vi "live view D05.vi"() -> ()   [LabVIEW 2019, in "D05.lvlib"]
uses:
  D05.lvlib
  <vilib>/userDefined/High Color/IMAQdx.ctl
  <vilib>/vision/Image Controls.llb/IMAQ Image.ctl
  <vilib>/measure/mamon.llb/Trigger Detection for 1 Channel.vi
  <vilib>/measure/NI_MAPro.lvlib
  Calibration Lib.lvlib
  database.lvlib
  <vilib>/vision/driver/NI_Vision_Acquisition_Software.lvlib
panel:
  out "Error out":errorcluster
  in  "Save Button":bool
  in  "Calib IMQ Num":u16(ring) items=["First IMQ", "Second IMQ", "Third IMQ"]
  in  "Verify Calibration1 D05":bool caption="capture grab"
  in  "snapshot":bool
  out "error prj04":errorcluster
  in  "Verify Calibration D05":bool caption="capture grab"
  in  "Close":bool
  in  "Method 2 save D05":bool caption="capture grab"
  in  "Method 1 Save D05":bool caption="Saving txt"
  out "Average Result":string="Average Result"
  out ">18  A":dbl(slide)=1.0 caption=">16 mm" scale=0.0..100.0
  out "16-18  A":dbl(slide)=1.0 caption="14-16 mm" scale=0.0..100.0
  out "14-16  A":dbl(slide)=1.0 caption="12.7-14 mm" scale=0.0..100.0
  out "12.5-14 A":dbl(slide)=1.0 caption="11-12.7 mm" scale=0.0..100.0
  out "10-12.5  A":dbl(slide)=1.0 caption="9.5-11 mm" scale=0.0..100.0 scale format="%#_4f"
  out "8-10  A":dbl(slide)=1.0 caption="8-9.5 mm" scale=0.0..100.0
  out "6.3-8  A":dbl(slide)=1.0 caption="6.3-8 mm" scale=0.0..100.0
  out "<6.3  A":dbl(slide)=1.0 caption="<6.3 mm" scale=0.0..100.0
  out "Live Result":string="Live Result"
  out ">18  L":dbl(slide)=1.0 caption=">16 mm" scale=0.0..100.0
  out "Live View":T1(plugin-control) caption="Disc 26"
  out "16-18  L":dbl(slide)=1.0 caption="14-16 mm" scale=0.0..100.0
  out "14-16  L":dbl(slide)=1.0 caption="12.7-14 mm" scale=0.0..100.0
  out "12.5-14 L":dbl(slide)=1.0 caption="11-12.7 mm" scale=0.0..100.0
  out "10-12.5  L":dbl(slide)=1.0 caption="9.5-11 mm" scale=0.0..100.0 scale format="%#_4f"
  out "8-10  L":dbl(slide)=1.0 caption="8-9.5 mm" scale=0.0..100.0
  out "6.3-8  L":dbl(slide)=1.0 caption="6.3-8 mm" scale=0.0..100.0
  out "<6.3  L":dbl(slide)=1.0 caption="<6.3 mm" scale=0.0..100.0
  out "disc name":string="Live Info Disc 05"
  out "dsgs":string="DSGS"
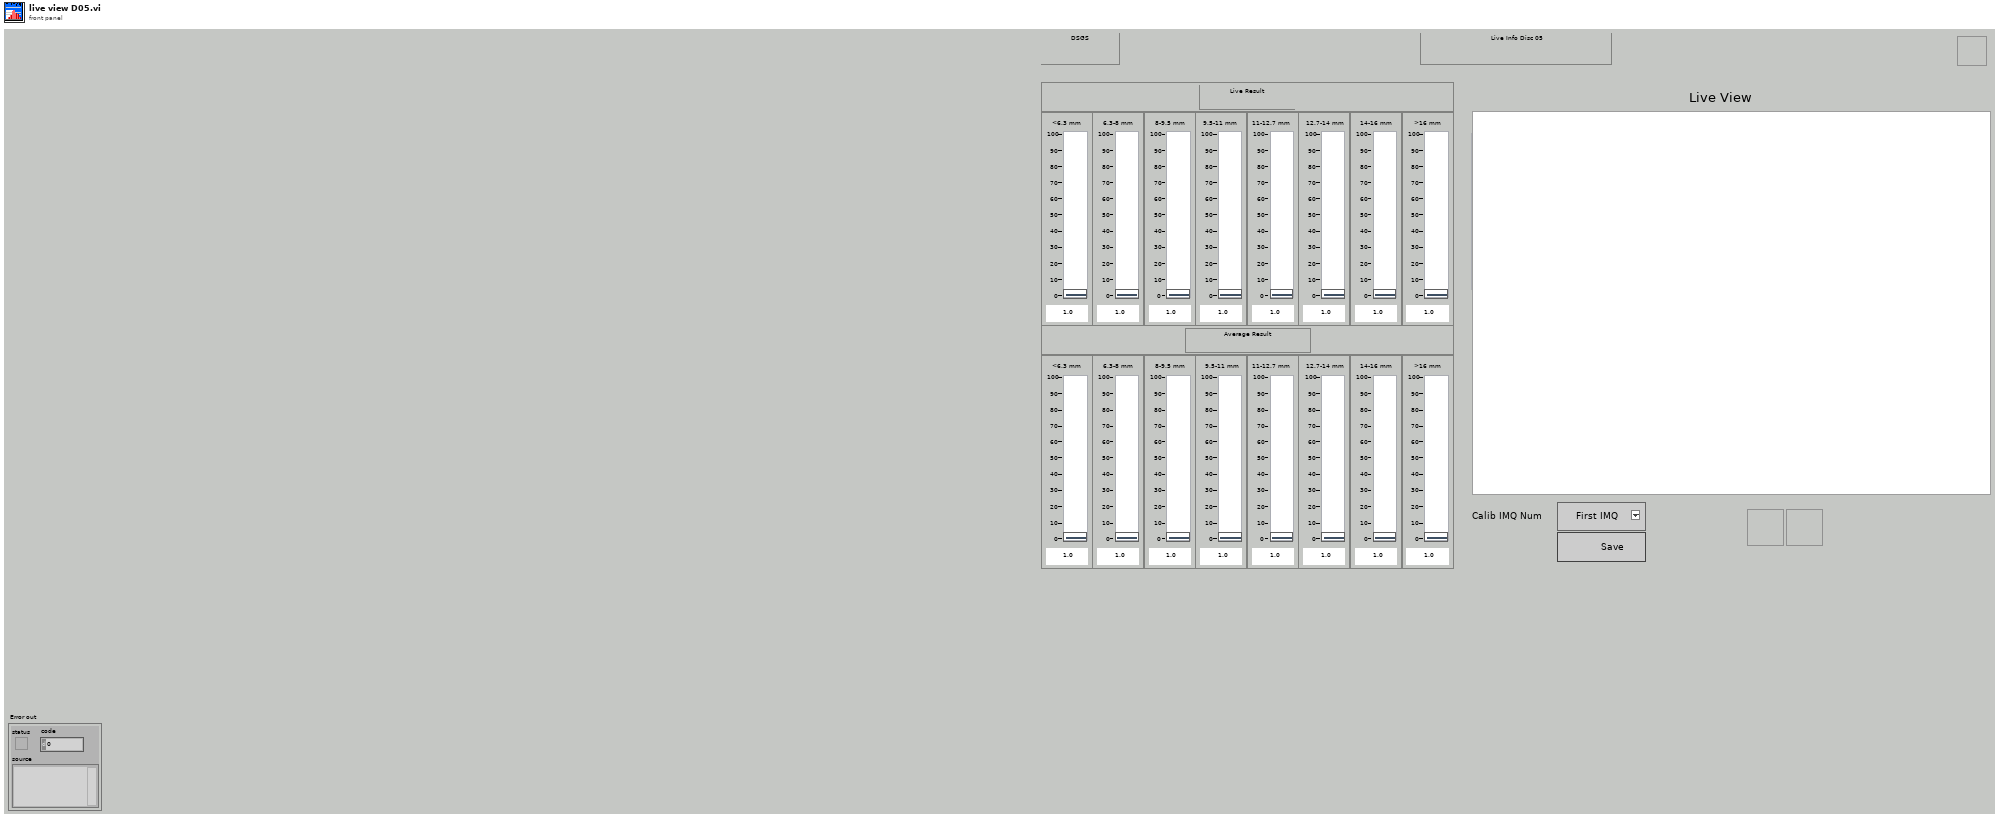
[diagram p1: front panel]
types:
  T1 = typedef "IMAQ Image.ctl" = refnum<image>
  T2 = typedef "IMAQdx.ctl" = refnum<k21>
  T3 = enum8{"Enabled", "Disabled", "Disabled and Grayed Out"}
  T4 = cluster{"date/time string":string, "date/time string":string, string, "Value":dbl, "Value":dbl, "Value":dbl, "Value":dbl, "Value":dbl, "Value":dbl, "Value":dbl, "Value":dbl}
  T5 = cluster{"date/time string":string, "date/time string":string, i32, "spreadsheet string":string, "spreadsheet string":string}
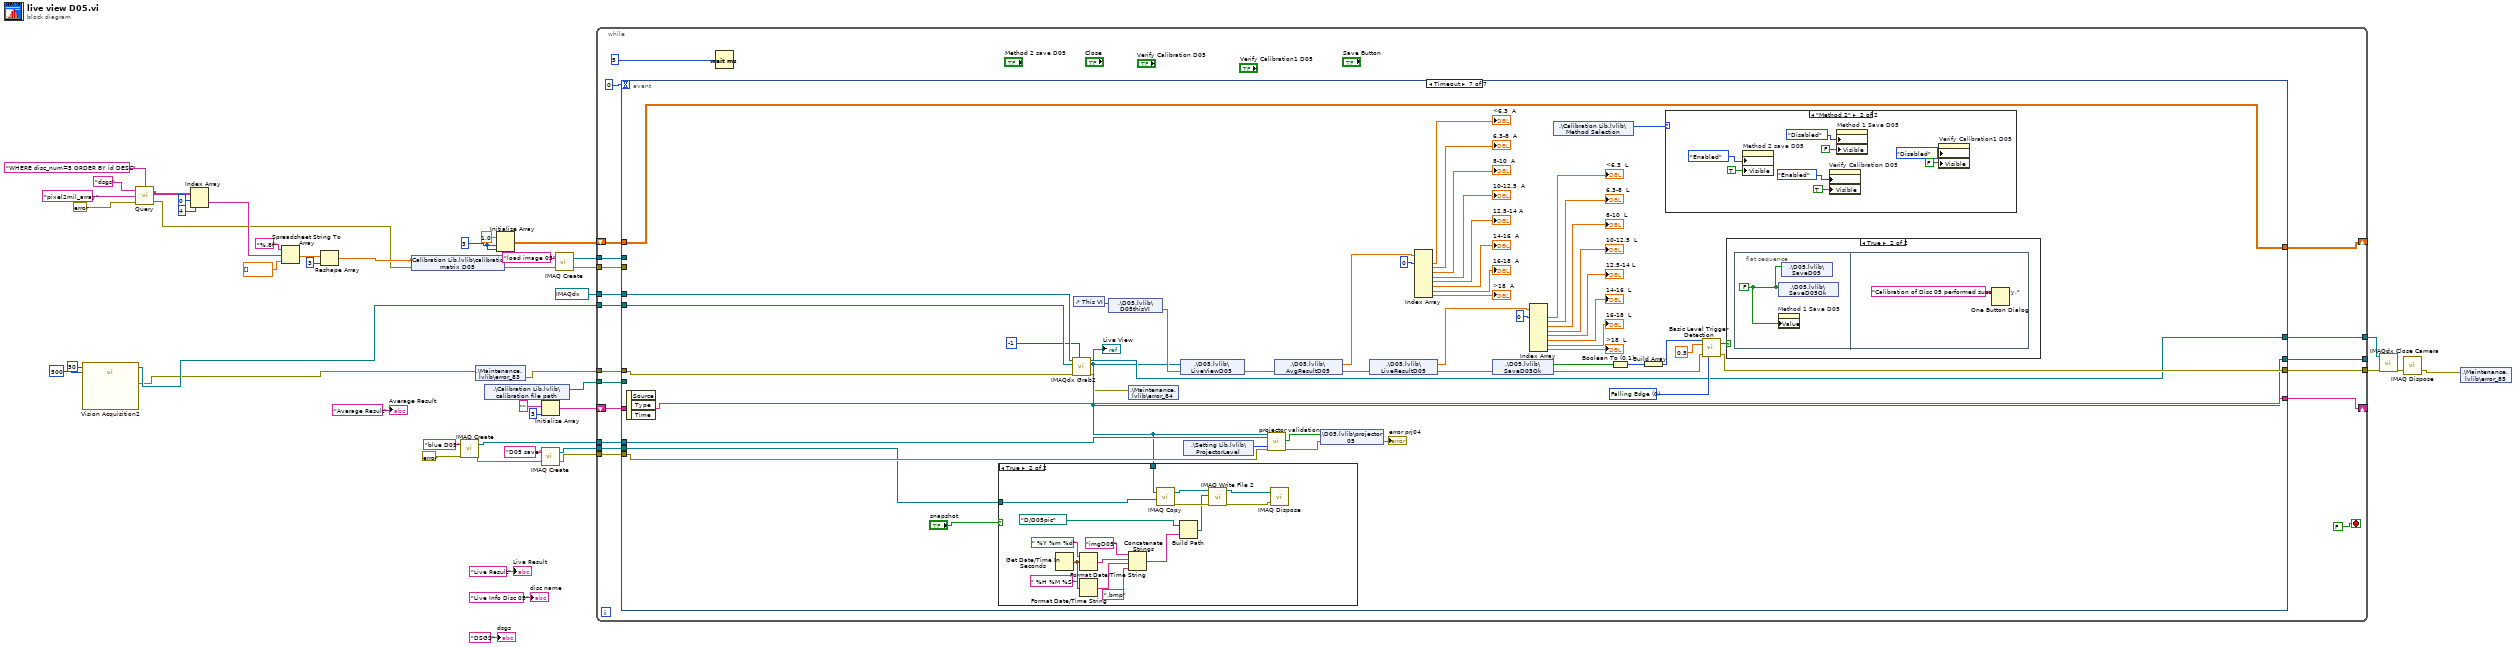
[diagram p0: block diagram]
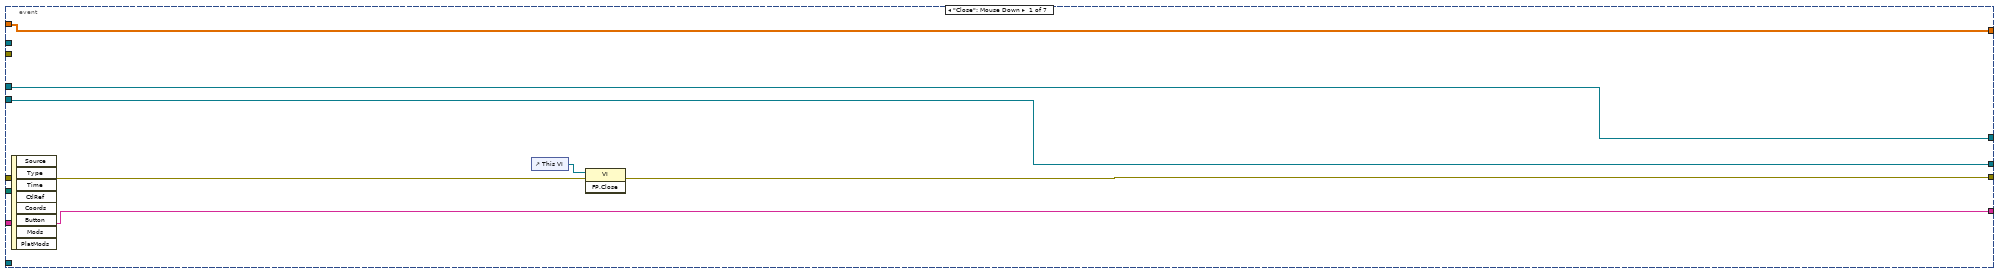
[diagram p2: hidden frame]
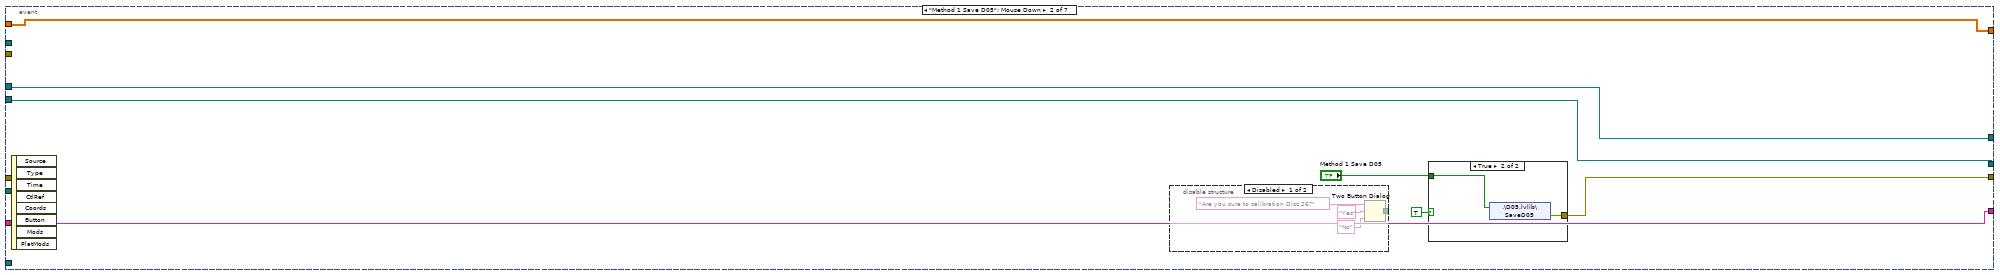
[diagram p3: hidden frame]
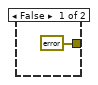
[diagram p5: hidden frame]
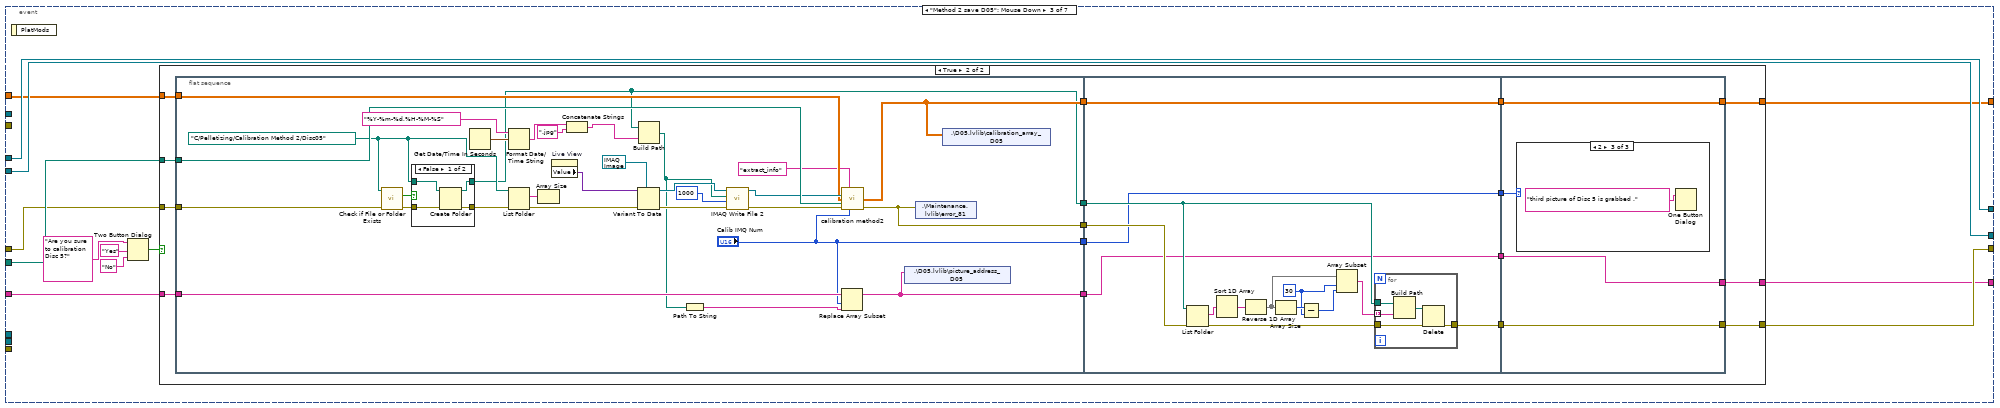
[diagram p6: hidden frame]
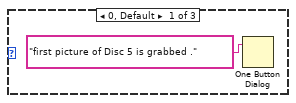
[diagram p9: hidden frame]
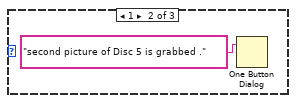
[diagram p10: hidden frame]
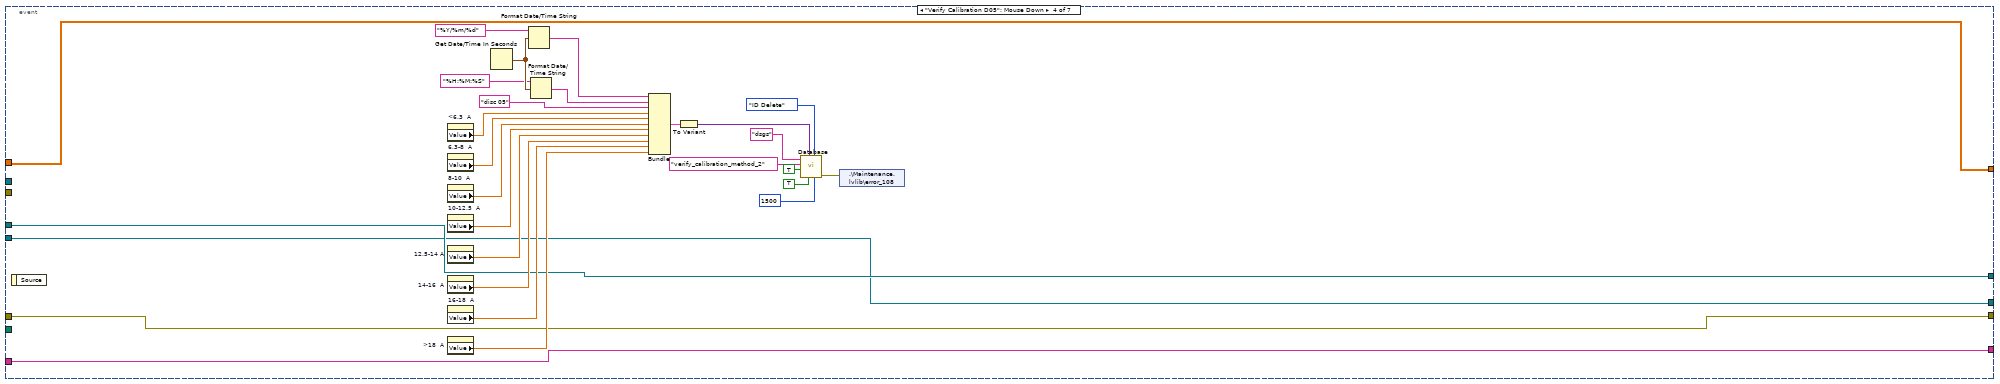
[diagram p11: hidden frame]
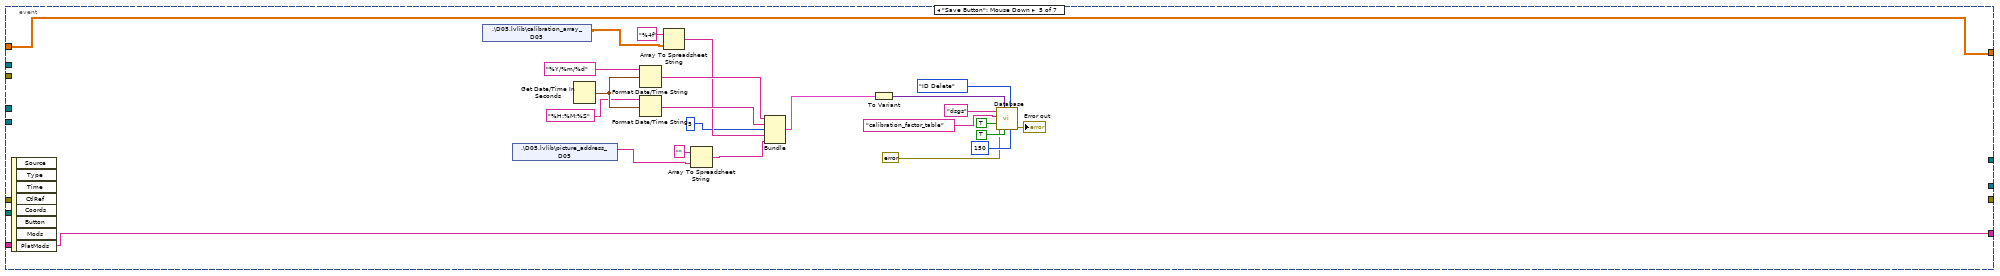
[diagram p12: hidden frame]
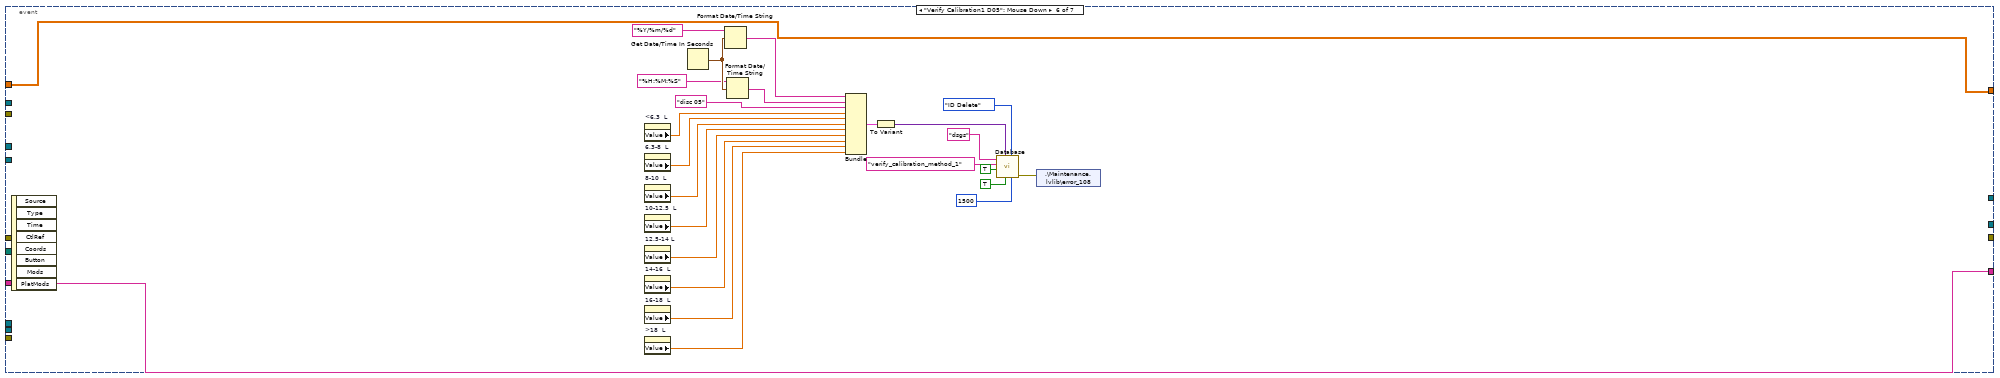
[diagram p13: hidden frame]
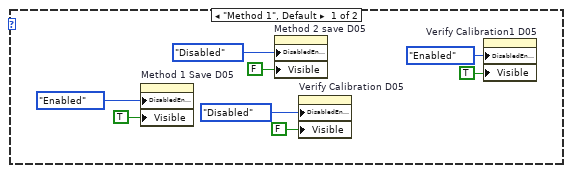
[diagram p15: hidden frame]
diagram:
  w15 = 3 ("dimension size")
  n1 = call "Vision Acquisition2"("Gain (Raw)"=i64 50, "Exposure Time (Raw)"=i64 500) -> ("Image Out"=w4:T1, "error out"=w3:errorcluster)  [unwired: 23 in, 1 out]
  n2 = call "Query.vi"("Condition"="WHERE disc_num=5 ORDER BY id DESC", "Error in"=errorcluster {"status"=FALSE, "code"=0, "source"=""}, "Table Name"="pixel2mil_array", "Connection Name"="dsgs") -> ("Error out"=w7:errorcluster, "data"=w10:string[][])
  n3 = Index Array(array=w10, index (row)=0, index (col)=4 ("disabled index (col)")) -> (element=w8:string)
  n4 = Spreadsheet String To Array(format string="%.8f", spreadsheet string=w8, array type (2D Dbl)=sgl[] []) -> (array=w28:sgl[])  [unwired: 1 in]
  n5 = Reshape Array(w28, 3 ("dimension size")) -> (w25:sgl[])
  n6 = shared-variable ".\\Calibration Lib.lvlib\\calibration matrix D05"(w25, error in=w7) -> (error out=w24:errorcluster)
  n7 = call "IMAQ Create"("Image Name"="blue D05", "error in (no error)"=errorcluster {"status"=FALSE, "code"=0, "source"=""}) -> ("New Image"=w22:T1, "error out"=w20:errorcluster)  [unwired: 3 in]
  n8 = shared-variable ".\\Maintenance.lvlib\\error_83"(w3) -> (error out=w37:errorcluster)  [unwired: 1 in]
  n9 = shared-variable ".\\Calibration Lib.lvlib\\calibration file path"() -> (w38:path)  [unwired: 1 in, 1 out]
  n10 = Initialize Array(1.0 ("element"), w15, w15) -> (w14:dbl[][])
  n11 = call "IMAQ Create"("Image Name"="D05 save", "error in (no error)"=w20) -> ("New Image"=w17:T1, "error out"=w19:errorcluster)  [unwired: 3 in]
  n12 = Initialize Array("", 3 ("dimension size")) -> (w11:string[])
  n13 = call "IMAQ Create"("Image Name"="load image 05", "error in (no error)"=w24) -> ("New Image"=w34:T1, "error out"=w35:errorcluster)  [unwired: 3 in]
  n14 = while {
    tunnel: w38 -> [w63]
    tunnel: w37 -> [w62]
    tunnel: w4 -> [w60]
    tunnel: [w59] -> w42
    tunnel: [w58] -> _
    tunnel: T2 "cam4" ("Session In") -> [w57]
    tunnel: [w56] -> w39
    tunnel: w35 -> [w55]
    tunnel: w34 -> [w54]
    tunnel: w22 -> [w53]
    tunnel: w19 -> [w52]
    tunnel: w17 -> [w51]
    shift-right: [w49] -> _
    shift-left: w14 -> [w50]
    shift-right: [w47] -> _
    shift-left: w11 -> [w48]
    stop <- FALSE stop-if-true
    n15 = event shown="[6] Timeout" {
      selector: _ -> [_ _ _ _ _ _ _]
      dyn-events: _ -> [_ _ _ _ _ _ _]
      timeout: 0 -> [_ _ _ _ _ _ _]
      tunnel: w63 -> [_ _ w99 _ _ _ _]
      tunnel: [w71 w79 w95 w187 _ _ w276] -> w59
      tunnel: w62 -> [w70 _ w98 w187 _ _ w259]
      tunnel: w60 -> [w69 w78 w97 w185 _ _ w264]
      tunnel: [w69 w78 w97 w185 _ _ w261] -> w58
      tunnel: w57 -> [w68 w77 w96 w186 _ _ w263]
      tunnel: [w68 w77 w96 w186 _ _ w262] -> w56
      tunnel: w55 -> [_ _ _ _ _ _ _]
      tunnel: w54 -> [_ _ _ _ _ _ _]
      tunnel: w53 -> [_ _ _ _ _ _ w274]
      tunnel: w52 -> [_ _ _ _ _ _ w270]
      tunnel: w51 -> [_ _ _ _ _ _ w267]
      tunnel: w50 -> [w67 w74 w90 w182 w211 w234 w266]
      tunnel: [w67 w74 w89 w182 w211 w234 w266] -> w49
      tunnel: w48 -> [w66 w73 w88 w181 w210 w233 w265]
      tunnel: [w66 w73 w87 w181 w210 w233 w265] -> w47
      event "Close": Mouse Down {
        n16 = event-data() -> ()  [unwired: 1 in, 8 out]
        n17 = control-ref of="This VI"() -> (w72:refnum<vi>)
        n18 = invoke class="VI" method="FP.Close"(reference=w72, error in=w70) -> (error out=w71:errorcluster)  [unwired: 1 in, 2 out]
      }
      event "Method 1 Save D05": Mouse Down {
        n19 = event-data() -> ()  [unwired: 1 in, 8 out]
        n20 = disable-structure shown="Disabled" {
          disable-tunnel: [w80 _] -> _
          frame Disabled {
            n21 = Two Button Dialog(message="Are you sure to calibration Disc 26?", 1:"No" ("F button name (\"Cancel\")"), 2:"Yes" ("T button name (\"OK\")")) -> (T button?=w80:bool)
          }
          frame Enabled {
          }
        }
        n22 = case shown="True" TRUE {
          tunnel: [errorcluster {"status"=FALSE, "code"=0, "source"=""} ("error IO") w86] -> w79
          tunnel: "Method 1 Save D05" -> [_ w85]
          frame False {
          }
          frame True {
            n23 = shared-variable ".\\D05.lvlib\\SaveD05"(w85) -> (error out=w86:errorcluster)  [unwired: 1 in]
          }
        }
      }
      event "Method 2 save D05": Mouse Down {
        n24 = event-data() -> ()  [unwired: 1 in, 1 out]
        n25 = Two Button Dialog(message="Are you sure to calibration Disc 5?", 1:"No" ("F button name (\"Cancel\")"), 2:"Yes" ("T button name (\"OK\")")) -> (T button?=w91:bool)
        n26 = case shown="True" w91 {
          tunnel: w99 -> [_ w117]
          tunnel: w98 -> [w102 w116]
          tunnel: [w102 w115] -> w95
          tunnel: w90 -> [w101 w113]
          tunnel: [w101 w110] -> w89
          tunnel: w88 -> [w100 w109]
          tunnel: [w100 w106] -> w87
          frame False {
          }
          frame True {
            n27 = flat-sequence {
              tunnel: w116 -> [w137]
              tunnel: w117 -> [w148]
              tunnel: [w123] -> w118
              tunnel: w113 -> [w130]
              tunnel: [w129] -> w111
              tunnel: w109 -> [w126]
              tunnel: [w125] -> w107
              tunnel: [w124] -> w105
              tunnel: ["Calib IMQ Num"] -> w103
              tunnel: [w159] -> w114
              tunnel: [w157] -> w112
              tunnel: [w156] -> w108
              tunnel: w105 -> [w160]
              tunnel: w107 -> [w156]
              tunnel: w111 -> [w157]
              tunnel: w118 -> [w161]
              tunnel: [w155] -> w104
              tunnel: w103 -> [w155]
              tunnel: [w177] -> w115
              tunnel: w114 -> [w177]
              tunnel: [w176] -> w110
              tunnel: w112 -> [w176]
              tunnel: [w175] -> w106
              tunnel: w108 -> [w175]
              tunnel: w104 -> [w174]
              frame #0 {
                w133 = path "C:/Pelletizing/Calibration Method 2/Disc05" ("path")
                n28 = call <vilib>:"Check if File or Folder Exists.vi"("error in (no error)"=w137, "path"=w133) -> ("error out"=w138:errorcluster, "file or folder exists?"=w139:bool)  [unwired: 7 in, 1 out]
                n29 = case shown="False" w139 {
                  tunnel: [w150 w154] -> w123
                  tunnel: w133 -> [w152 w154]
                  tunnel: w138 -> [w151 w153]
                  tunnel: [w149 w153] -> w135
                  frame False {
                    n30 = Create Folder(path (use dialog)=w152, error in=w151) -> (created path=w150:path, error out=w149:errorcluster)  [unwired: 1 in, 1 out]
                  }
                  frame True {
                  }
                }
                n31 = Get Date/Time In Seconds() -> (seconds since 1Jan1904=w143:timestamp)
                n32 = Format Date/Time String(time format string (%c)="%Y-%m-%d,%H-%M-%S", seconds (now)=w143) -> (date/time string=w141:string)  [unwired: 1 in]
                n33 = List Folder(path=w133, error in=w135) -> (filenames=w136:string[], error out=w134:errorcluster)  [unwired: 2 in, 2 out]
                n34 = Array Size(array=w136) -> ()  [unwired: 1 out]
                n35 = property on="Live View" class="ImageControl"() -> ("Value"=w147:variant)  [unwired: 2 in, 2 out]
                n36 = Concatenate Strings(w141, ".jpg" ("string")) -> (w122:string)
                n37 = Variant To Data(error in=w134, type=T1 refnum ("New Image"), Variant=w147) -> (data=w131:T1, error out=w144:errorcluster)
                n38 = Build Path(base path=w123, name or relative path=w122) -> (appended path=w121:path)
                n39 = Path To String(path=w121) -> (string=w120:string)
                n40 = call-poly "IMAQ Write File 2"("error in (no error)"=w144, "Image Quality"=u32 1000, "File Path"=w121, "Image"=w131) -> ("error out"=w128:errorcluster, "Image Out (duplicate)"=w132:T1)  [unwired: 6 in]
                n41 = Replace Array Subset(array=w126, new element=w120, index="Calib IMQ Num") -> (w125:string[])
                n42 = call "calibration method2.vi"("function name"="extract_info", "Image IN"=w132, "initialize matrix"=w130, "module path"=w148, "error in"=w128, "snap number"="Calib IMQ Num") -> ("calibration matrix"=w129:dbl[][], "error out"=w124:errorcluster)  [unwired: 8 in]
                n43 = shared-variable ".\\D05.lvlib\\picture_address_D05"(w125) -> ()  [unwired: 1 in, 1 out]
                n44 = shared-variable ".\\Maintenance.lvlib\\error_81"(w124) -> ()  [unwired: 1 in, 1 out]
                n45 = shared-variable ".\\D05.lvlib\\calibration_array_D05"(w129) -> ()  [unwired: 1 in, 1 out]
              }
              frame #1 {
                w162 = 30 ("index")
                n46 = List Folder(path=w161, error in=w160) -> (filenames=w168:string[], error out=w158:errorcluster)  [unwired: 2 in, 2 out]
                n47 = Sort 1D Array(array=w168) -> (sorted array=w167:string[])
                n48 = Reverse 1D Array(array=w167) -> (reversed array=w166:string[])
                n49 = Array Size(array=w166) -> (size(s)=w165:i32)
                n50 = Subtract(x=w165, y=w162) -> (x-y=w164:i32)
                n51 = Array Subset(array=w166, index=w162, length=w164) -> (w163:string[])
                n52 = for {
                  tunnel: w163 -> [w172] mode=indexing
                  tunnel: w161 -> [w173]
                  tunnel: [w170] -> w159
                  tunnel: w158 -> [w169]
                  n53 = Build Path(base path=w173, name or relative path=w172) -> (appended path=w171:path)
                  n54 = Delete(path (use dialog)=w171, error in=w169) -> (error out=w170:errorcluster)  [unwired: 3 in, 2 out]
                }
              }
              frame #2 {
                n55 = case shown="2" w174 {
                  frame 0, Default {
                    n56 = One Button Dialog(message="first picture of Disc 5 is grabbed .") -> ()  [unwired: 1 in, 1 out]
                  }
                  frame 1 {
                    n57 = One Button Dialog(message="second picture of Disc 5 is grabbed .") -> ()  [unwired: 1 in, 1 out]
                  }
                  frame 2 {
                    n58 = One Button Dialog(message="third picture of Disc 5 is grabbed .") -> ()  [unwired: 1 in, 1 out]
                  }
                }
              }
            }
          }
        }
      }
      event "Verify Calibration D05": Mouse Down {
        n59 = event-data() -> ()  [unwired: 1 in, 1 out]
        n60 = property on="<6.3  A" class="Slide (strict)"() -> ("Value"=w202:dbl)  [unwired: 2 in, 2 out]
        n61 = property on="6.3-8  A" class="Slide (strict)"() -> ("Value"=w201:dbl)  [unwired: 2 in, 2 out]
        n62 = property on="8-10  A" class="Slide (strict)"() -> ("Value"=w200:dbl)  [unwired: 2 in, 2 out]
        n63 = property on="10-12.5  A" class="Slide (strict)"() -> ("Value"=w199:dbl)  [unwired: 2 in, 2 out]
        n64 = property on="12.5-14 A" class="Slide (strict)"() -> ("Value"=w198:dbl)  [unwired: 2 in, 2 out]
        n65 = property on="14-16  A" class="Slide (strict)"() -> ("Value"=w197:dbl)  [unwired: 2 in, 2 out]
        n66 = property on="16-18  A" class="Slide (strict)"() -> ("Value"=w196:dbl)  [unwired: 2 in, 2 out]
        n67 = property on=">18  A" class="Slide (strict)"() -> ("Value"=w195:dbl)  [unwired: 2 in, 2 out]
        n68 = Get Date/Time In Seconds() -> (seconds since 1Jan1904=w207:timestamp)
        n69 = Format Date/Time String(time format string (%c)="%Y/%m/%d", seconds (now)=w207) -> (date/time string=w205:string)  [unwired: 1 in]
        n70 = Format Date/Time String(time format string (%c)="%H:%M:%S", seconds (now)=w207) -> (date/time string=w204:string)  [unwired: 1 in]
        n71 = Bundle("date/time string"=w205, "date/time string"=w204, "disc 05", "Value"=w202, "Value"=w201, "Value"=w200, "Value"=w199, "Value"=w198, "Value"=w197, "Value"=w196, "Value"=w195) -> (w194:T4)  [unwired: 1 in]
        n72 = To Variant(anything=w194) -> (Variant=w193:variant)
        n73 = call "Database.vi"("Maximum Row"=1500, "Enum"=enum16{"ID Delete", "Time Delete"}."ID Delete", "Delete row?"=TRUE, "Data"=w193, "Auto Increment ID?"=TRUE, "Table"="verify_calibration_method_2", "Connection"="dsgs") -> ("Error out"=w188:errorcluster)  [unwired: 4 in]
        n74 = shared-variable ".\\Maintenance.lvlib\\error_108"(w188) -> ()  [unwired: 1 in, 1 out]
      }
      event "Save Button": Mouse Down {
        n75 = event-data() -> ()  [unwired: 1 in, 8 out]
        n76 = shared-variable ".\\D05.lvlib\\calibration_array_D05"() -> (w212:dbl[][])  [unwired: 1 in, 1 out]
        n77 = shared-variable ".\\D05.lvlib\\picture_address_D05"() -> (w214:string[])  [unwired: 1 in, 1 out]
        n78 = Get Date/Time In Seconds() -> (seconds since 1Jan1904=w221:timestamp)
        n79 = Format Date/Time String(time format string (%c)="%Y/%m/%d", seconds (now)=w221) -> (date/time string=w222:string)  [unwired: 1 in]
        n80 = Format Date/Time String(time format string (%c)="%H:%M:%S", seconds (now)=w221) -> (date/time string=w220:string)  [unwired: 1 in]
        n81 = Array To Spreadsheet String(array=w212, 3:"%4f" ("format string")) -> (spreadsheet string=w216:string)  [unwired: 1 in]
        n82 = Array To Spreadsheet String(array=w214, 3:"" ("format string")) -> (spreadsheet string=w213:string)  [unwired: 1 in]
        n83 = Bundle("date/time string"=w222, "date/time string"=w220, 5, "spreadsheet string"=w216, "spreadsheet string"=w213) -> (w225:T5)  [unwired: 1 in]
        n84 = To Variant(anything=w225) -> (Variant=w232:variant)
        n85 = call "Database.vi"("Maximum Row"=150, "Enum"=enum16{"ID Delete", "Time Delete"}."ID Delete", "Delete row?"=TRUE, "Data"=w232, "Error in"=errorcluster {"status"=FALSE, "code"=0, "source"=""}, "Auto Increment ID?"=TRUE, "Table"="calibration_factor_table", "Connection"="dsgs") -> ("Error out"=→"Error out":errorcluster)  [unwired: 3 in]
      }
      event "Verify Calibration1 D05": Mouse Down {
        n86 = event-data() -> ()  [unwired: 1 in, 8 out]
        n87 = property on="<6.3  L" class="Slide (strict)"() -> ("Value"=w251:dbl)  [unwired: 2 in, 2 out]
        n88 = property on="6.3-8  L" class="Slide (strict)"() -> ("Value"=w250:dbl)  [unwired: 2 in, 2 out]
        n89 = property on="8-10  L" class="Slide (strict)"() -> ("Value"=w249:dbl)  [unwired: 2 in, 2 out]
        n90 = property on="10-12.5  L" class="Slide (strict)"() -> ("Value"=w248:dbl)  [unwired: 2 in, 2 out]
        n91 = property on="12.5-14 L" class="Slide (strict)"() -> ("Value"=w247:dbl)  [unwired: 2 in, 2 out]
        n92 = property on="14-16  L" class="Slide (strict)"() -> ("Value"=w246:dbl)  [unwired: 2 in, 2 out]
        n93 = property on="16-18  L" class="Slide (strict)"() -> ("Value"=w245:dbl)  [unwired: 2 in, 2 out]
        n94 = property on=">18  L" class="Slide (strict)"() -> ("Value"=w244:dbl)  [unwired: 2 in, 2 out]
        n95 = Get Date/Time In Seconds() -> (seconds since 1Jan1904=w256:timestamp)
        n96 = Format Date/Time String(time format string (%c)="%Y/%m/%d", seconds (now)=w256) -> (date/time string=w254:string)  [unwired: 1 in]
        n97 = Format Date/Time String(time format string (%c)="%H:%M:%S", seconds (now)=w256) -> (date/time string=w253:string)  [unwired: 1 in]
        n98 = Bundle("date/time string"=w254, "date/time string"=w253, "disc 05", "Value"=w251, "Value"=w250, "Value"=w249, "Value"=w248, "Value"=w247, "Value"=w246, "Value"=w245, "Value"=w244) -> (w243:T4)  [unwired: 1 in]
        n99 = To Variant(anything=w243) -> (Variant=w242:variant)
        n100 = call "Database.vi"("Maximum Row"=1500, "Enum"=enum16{"ID Delete", "Time Delete"}."ID Delete", "Delete row?"=TRUE, "Data"=w242, "Auto Increment ID?"=TRUE, "Table"="verify_calibration_method_1", "Connection"="dsgs") -> ("Error out"=w237:errorcluster)  [unwired: 4 in]
        n101 = shared-variable ".\\Maintenance.lvlib\\error_108"(w237) -> ()  [unwired: 1 in, 1 out]
      }
      event Timeout {
        w284 = u16 0 items=["Falling Edge", "Rising Edge"] ("trigger slope")
        n102 = event-data() -> ()  [unwired: 1 in, 3 out]
        n103 = call <vilib>:"IMAQdx Grab2.vi"("Timeout (ms)"=-1, "error in"=w259, "Image In"=w264, "Session In"=w263) -> ("error out"=w260:errorcluster, "Image Out"=w261:T1, "Session Out"=w262:T2)  [unwired: 4 in, 1 out]
        "Live View" <- w261
        n104 = case shown="True" "snapshot" {
          tunnel: w267 -> [_ w324]
          tunnel: w261 -> [_ w323]
          frame False {
          }
          frame True {
            n105 = Get Date/Time In Seconds() -> (seconds since 1Jan1904=w317:timestamp)
            n106 = Format Date/Time String(time format string (%c)=" %Y %m %d", seconds (now)=w317) -> (date/time string=w313:string)  [unwired: 1 in]
            n107 = Format Date/Time String(time format string (%c)=" %H %M %S", seconds (now)=w317) -> (date/time string=w312:string)  [unwired: 1 in]
            n108 = Concatenate Strings("imgD05" ("string"), w313, w312, ".bmp" ("string")) -> (w310:string)
            n109 = call "IMAQ Copy"("Image Dst"=w324, "Image Src"=w323) -> ("error out"=w321:errorcluster, "Image Dst Out"=w322:T1)  [unwired: 4 in]
            n110 = Build Path(base path=path "D:/D05pic" ("File Path"), name or relative path=w310) -> (appended path=w309:path)
            n111 = call-poly "IMAQ Write File 2"("error in (no error)"=w321, "File Path"=w309, "Image"=w322) -> ("error out"=w319:errorcluster, "Image Out (duplicate)"=w320:T1)  [unwired: 7 in]
            n112 = call "IMAQ Dispose"("Image"=w320, "error in (no error)"=w319) -> ()  [unwired: 4 in, 1 out]
          }
        }
        n113 = control-ref of="This VI"() -> (w279:refnum<vi>)
        n114 = shared-variable ".\\D05.lvlib\\D05thisVI"(w279) -> (error out=w275:errorcluster)  [unwired: 1 in]
        n115 = shared-variable ".\\Maintenance.lvlib\\error_84"(w260) -> ()  [unwired: 1 in, 1 out]
        n116 = shared-variable ".\\D05.lvlib\\LiveViewD05"(w261, error in=w275) -> (error out=w278:errorcluster)
        n117 = shared-variable ".\\Setting Lib.lvlib\\ProjectorLevel"() -> (w269:i32)  [unwired: 1 in, 1 out]
        n118 = call "projector validation.vi"("Image Src"=w261, "blue channel"=w274, "on/off level"=w269, "error in (no error)"=w270) -> ("on/off"=w273:bool, "error out"=w272:errorcluster)  [unwired: 14 in]
        n119 = shared-variable ".\\D05.lvlib\\AvgResultD05"(error in=w278) -> (w299:dbl[], error out=w281:errorcluster)
        n120 = shared-variable ".\\D05.lvlib\\projector 05"(w273, error in=w272) -> (error out=→"error prj04":errorcluster)
        n121 = shared-variable ".\\D05.lvlib\\LiveResultD05"(error in=w281) -> (w298:dbl[], error out=w280:errorcluster)
        n122 = Index Array(array=w299, index #1=0 ("index")) -> (element #1=→"<6.3  A":dbl, element #2=→"6.3-8  A":dbl, element #3=→"8-10  A":dbl, element #4=→"10-12.5  A":dbl, element #5=→"12.5-14 A":dbl, element #6=→"14-16  A":dbl, element #7=→"16-18  A":dbl, element #8=→">18  A":dbl)  [unwired: 7 in]
        n123 = shared-variable ".\\D05.lvlib\\SaveD05Ok"(error in=w280) -> (w285:bool, error out=w277:errorcluster)
        n124 = Index Array(array=w298, index #1=0 ("index")) -> (element #1=→"<6.3  L":dbl, element #2=→"6.3-8  L":dbl, element #3=→"8-10  L":dbl, element #4=→"10-12.5  L":dbl, element #5=→"12.5-14 L":dbl, element #6=→"14-16  L":dbl, element #7=→"16-18  L":dbl, element #8=→">18  L":dbl)  [unwired: 7 in]
        n125 = shared-variable ".\\Calibration Lib.lvlib\\Method Selection"() -> (w282:enum32{"Method 1", "Method 2"})  [unwired: 1 in, 1 out]
        n126 = Boolean To (0,1)(Boolean=w285) -> (0, 1=w288:i16)
        n127 = Build Array(w288) -> (w287:i16[])
        n128 = case shown="\"Method 2\"" w282 {
          frame "Method 1", Default {
            n129 = property on="Method 1 Save D05" class="Bool (strict)"("DisabledEnum"=T3."Enabled" ("Disabled"), "Visible"=TRUE) -> ()  [unwired: 2 in, 2 out]
            n130 = property on="Method 2 save D05" class="Bool (strict)"("DisabledEnum"=T3."Disabled" ("Disabled"), "Visible"=FALSE) -> ()  [unwired: 2 in, 2 out]
            n131 = property on="Verify Calibration D05" class="Bool (strict)"("DisabledEnum"=T3."Disabled" ("Disabled"), "Visible"=FALSE) -> ()  [unwired: 2 in, 2 out]
            n132 = property on="Verify Calibration1 D05" class="Bool (strict)"("DisabledEnum"=T3."Enabled" ("Disabled"), "Visible"=TRUE) -> ()  [unwired: 2 in, 2 out]
          }
          frame "Method 2" {
            n133 = property on="Method 2 save D05" class="Bool (strict)"("DisabledEnum"=T3."Enabled" ("Disabled"), "Visible"=TRUE) -> ()  [unwired: 2 in, 2 out]
            n134 = property on="Verify Calibration D05" class="Bool (strict)"("DisabledEnum"=T3."Enabled" ("Disabled"), "Visible"=TRUE) -> ()  [unwired: 2 in, 2 out]
            n135 = property on="Method 1 Save D05" class="Bool (strict)"("DisabledEnum"=T3."Disabled" ("Disabled"), "Visible"=FALSE) -> ()  [unwired: 2 in, 2 out]
            n136 = property on="Verify Calibration1 D05" class="Bool (strict)"("DisabledEnum"=T3."Disabled" ("Disabled"), "Visible"=FALSE) -> ()  [unwired: 2 in, 2 out]
          }
        }
        n137 = call-poly <vilib>:"Basic Level Trigger Detection.vi"("signal in"=w287, "level"=0.5, "error in (no error)"=w277, "trigger slope"=w284) -> ("trigger detected?"=w283:bool, "error out"=w276:errorcluster)  [unwired: 9 in, 1 out]
        n138 = case shown="True" w283 {
          frame False {
          }
          frame True {
            n139 = flat-sequence {
              frame #0 {
                w341 = FALSE
                n140 = shared-variable ".\\D05.lvlib\\SaveD05Ok"(w341) -> ()  [unwired: 1 in, 1 out]
                n141 = property on="Method 1 Save D05" class="Bool (strict)"("Value"=w341) -> ()  [unwired: 2 in, 2 out]
                n142 = shared-variable ".\\D05.lvlib\\SaveD05"(w341) -> ()  [unwired: 1 in, 1 out]
              }
              frame #1 {
                n143 = One Button Dialog(message="Calibration of Disc 05 performed successfully.") -> ()  [unwired: 1 in, 1 out]
              }
            }
          }
        }
      }
    }
    n144 = Wait (ms)(milliseconds to wait=u32 5) -> ()  [unwired: 1 out]
  }
  n145 = call <vilib>:"IMAQdx Close Camera.vi"("error in"=w42, "Session In"=w39) -> ("error out"=w41:errorcluster)  [unwired: 9 in]
  n146 = call "IMAQ Dispose"("error in (no error)"=w41) -> ("error out"=w5:errorcluster)  [unwired: 5 in]
  n147 = shared-variable ".\\Maintenance.lvlib\\error_85"(w5) -> ()  [unwired: 1 in, 1 out]
  "Live Result" <- "Live Result" ("Live Result")
  "Average Result" <- "Average Result" ("Average Result")
  "disc name" <- "Live Info Disc 05" ("Live Result")
  "dsgs" <- "DSGS" ("Live Result")
